vi "Thermocouple Simulation PointByPoint.vi"() -> ()   [LabVIEW 8.6]
uses:
  vi.lib/UeiDaq/UeiDaqConfigureTimingForSimpleIO.vi
  vi.lib/UeiDaq/UeiDaqReadOneScaledScan.vi
  vi.lib/UeiDaq/UeiDaqWriteOneScaledScan.vi
  vi.lib/UeiDaq/UeiDaqCreateTCSession.vi
  <libdir>/resource/objmgr/UeiDaq.rc
panel:
  out "CJC temperature":dbl[](array[numeric])
  in  "Temperature Scale":i32(ring) items=["Celsius", "Fahrenheit", "Kelvin", "Rankine"]
  in  "Thermocouple type":i32(ring) items=["Type E", "Type J", "Type K", "Type R", "Type S", "Type T", "Type B", "Type N", "Type C"]
  in  "Output Values":dbl[](array[numeric])
  in  "AO Resource":string
  out "Waveform Chart":dbl[][](graph)
  in  "Refresh rate (ms)":u32
  in  "stop":bool
  in  "Diag Resource":string
  # "Simulate TC on TC-378 and read-back using diagnostic channels"
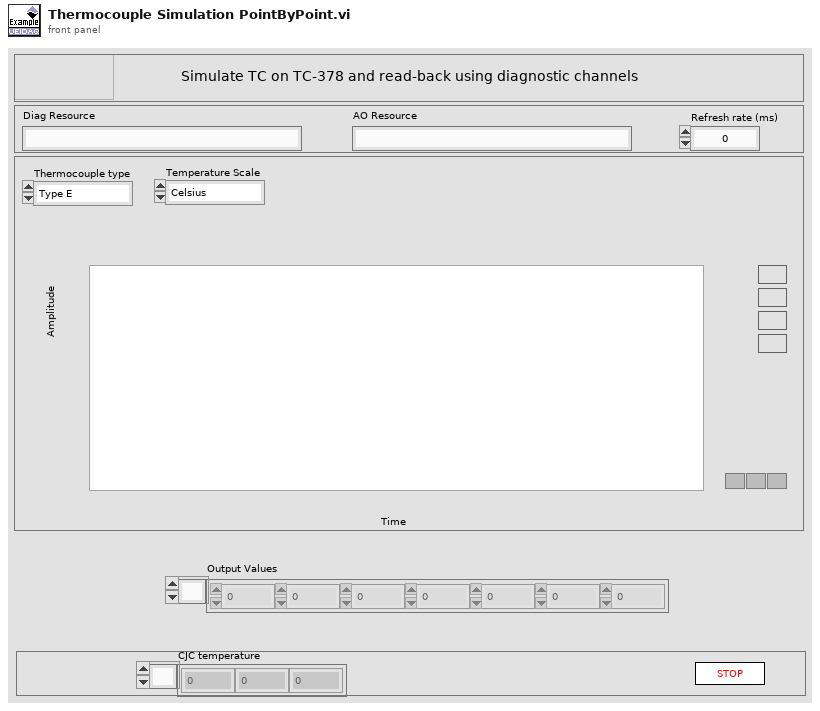
[diagram p1: front panel]
types:
  T1 = cluster{"Cold Junction compensation type":i32, "Cold Junction Compensationtemperature":dbl, "Cold Junction Compensation channel":string}
  T2 = cluster{"Thermocouple type":i32, "Temperature Scale":i32}
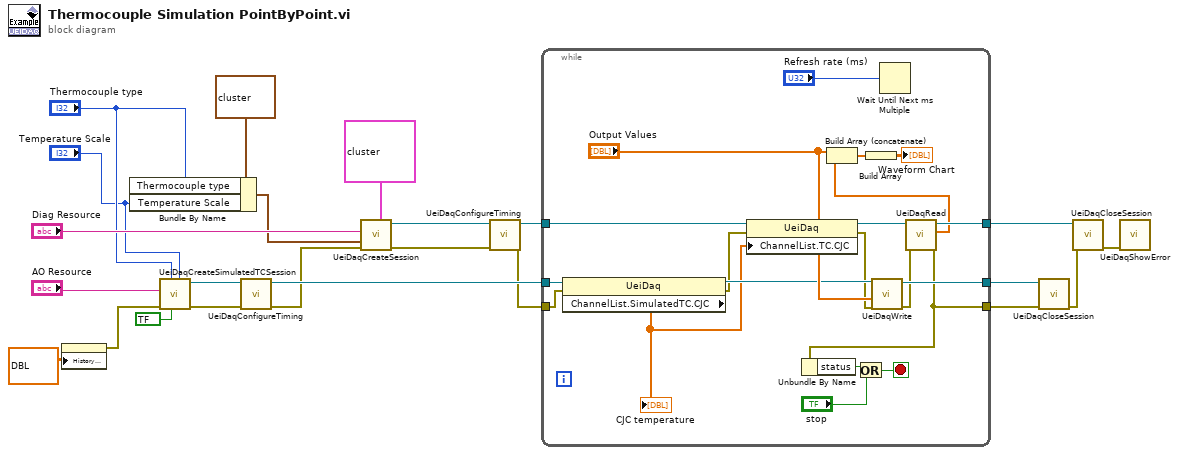
[diagram p0: block diagram]
diagram:
  n1 = property on="Waveform Chart" class="WFChart (strict)"("History Data"=dbl[][] ?) -> (error out=w9:errorcluster)  [unwired: 2 in, 1 out]
  n2 = Bundle By Name(cluster=T2 ? ("TC settings"), "Thermocouple type"="Thermocouple type", "Temperature Scale"="Temperature Scale") -> (w7:T2)
  n3 = call "UeiDaqCreateSimulatedTCSession.vi"("Temperature Scale"="Temperature Scale", "CJC enabled"=bool ?, "Thermocouple type"="Thermocouple type", "error in (no error)"=w9, "Resource"="AO Resource") -> ("error out"=w21:errorcluster, "UeiDaq Refnum Out"=w22:refnum<k20>)  [unwired: 5 in]
  n4 = call-poly "UeiDaqConfigureTiming.vi"("error in (no error)"=w21, "UeiDaq Refnum In"=w22) -> ("error out"=w15:errorcluster, "UeiDaq Refnum Out"=w20:refnum<k20>)  [unwired: 8 out]
  n5 = call-poly "UeiDaqCreateSession.vi"("Cold Junction Compensation Settings"=T1 ?, "error in (no error)"=w15, "TC settings"=w7, "Resource"="Diag Resource") -> ("error out"=w1:errorcluster, "UeiDaq Refnum Out"=w2:refnum<k20>)  [unwired: 4 in, 2 out]
  n6 = call-poly "UeiDaqConfigureTiming.vi"("error in (no error)"=w1, "UeiDaq Refnum In"=w2) -> ("error out"=w16:errorcluster, "UeiDaq Refnum Out"=w17:refnum<k20>)  [unwired: 8 out]
  n7 = while {
    tunnel: w20 -> [w32]
    tunnel: [w41] -> w23
    tunnel: w17 -> [w28]
    tunnel: w16 -> [w30]
    tunnel: [w39] -> w14
    tunnel: [w34] -> w13
    stop <- w42 stop-if-true
    n8 = property class="UeiDaq"(reference=w32, error in=w30) -> (reference out=w31:refnum<k20>, error out=w26:errorcluster, "ChannelList.SimulatedTC.CJC"=w27:dbl[])
    "CJC temperature" <- w27
    n9 = property class="UeiDaq"(reference=w28, error in=w26, "ChannelList.TC.CJC"=w27) -> (reference out=w29:refnum<k20>, error out=w25:errorcluster)
    n10 = call-poly "UeiDaqWrite.vi"("error in (no error)"=w25, "Scaled Data"="Output Values", "UeiDaq Refnum In"=w31) -> ("error out"=w24:errorcluster, "UeiDaq Refnum Out"=w41:refnum<k20>)  [unwired: 1 in, 6 out]
    n11 = Wait Until Next ms Multiple(millisecond multiple="Refresh rate (ms)") -> ()  [unwired: 1 out]
    n12 = call-poly "UeiDaqRead.vi"("error in (no error)"=w24, "UeiDaq Refnum In"=w29) -> ("error out"=w34:errorcluster, "Scaled Data"=w37:dbl[], "UeiDaq Refnum Out"=w39:refnum<k20>)  [unwired: 7 out]
    n13 = Unbundle By Name(w34) -> ("status"=w38:bool)
    n14 = Build Array (concatenate)("Output Values", w37) -> (w36:dbl[])
    n15 = Or(x=w38, y="stop") -> (x .or. y?=w42:bool)
    n16 = Build Array(w36) -> (→"Waveform Chart":dbl[][])
  }
  n17 = call "UeiDaqCloseSession.vi"("error in (no error)"=w13, "UeiDaq Refnum In"=w23) -> ("error out"=w12:errorcluster)  [unwired: 1 in, 8 out]
  n18 = call "UeiDaqCloseSession.vi"("error in (no error)"=w12, "UeiDaq Refnum In"=w14) -> ("error out"=w11:errorcluster)  [unwired: 1 in, 8 out]
  n19 = call "UeiDaqShowError.vi"("error in (no error)"=w11) -> ()  [unwired: 2 in, 9 out]
